vi "GW_Search_id.vi"(8 "error in (no error)":errorcluster, 10 "id":i16, 11 "DBlink":string="Driver={ODBC Driver 17 for SQL Server};Server=localhost\\SQLEXPRESS;Database=ZDX201;UID=labview;PWD=Dsa@54137926") -> (0 "error out":errorcluster, 1 "[glue_data_id]":string, 2 "找到":bool, 3 "取得ID":i16)   [LabVIEW 2019]
uses:
  <vilib>/addons/database/Connection.llb/DB Tools Open Connec (String).vi
  <vilib>/addons/database/Connection.llb/Conn Execute.vi
  <vilib>/addons/database/Recordset.llb/Rec Fetch Recordset Data (R).vi
  <vilib>/addons/database/Recordset.llb/Rec Destroy - Connection.vi
  <vilib>/addons/database/_DB Variant To Data/Database Variant To Data.xnode
  <vilib>/addons/database/NI_Database_API.lvlib
panel:
  out "size(s)":i32
  out "查詢結果":string="SELECT \n      [glue_data_id]\n  FROM [ZDX201].[dbo].[glue_workspace]\n where  [glue_data_id] is not null  and  [id]=0"
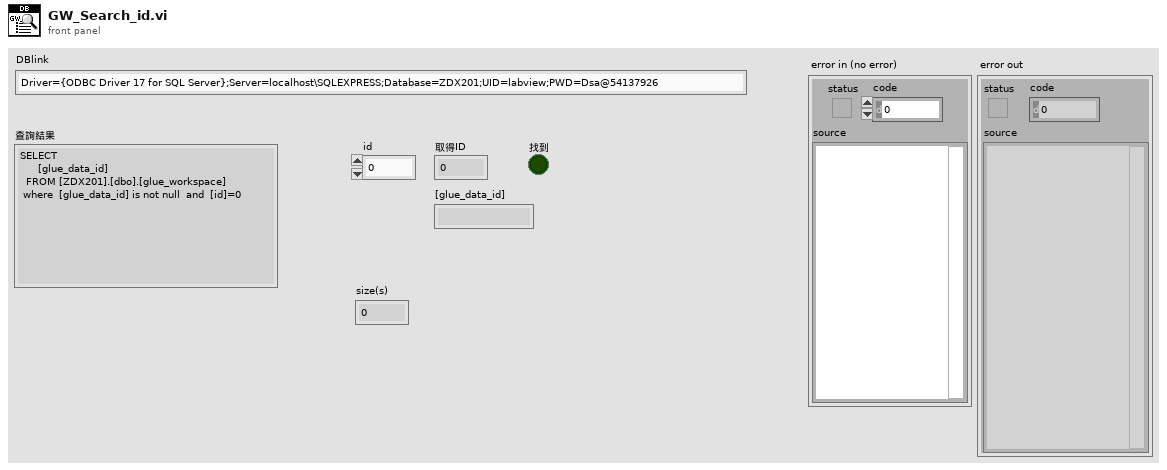
[diagram p1: front panel]
types:
  T1 = typedef "NI_Database_API.lvlib/Conn ObjectReference.ctl" = refnum<k1>
  T2 = typedef "NI_Database_API.lvlib/Rec ObjectReference.ctl" = refnum<k1>
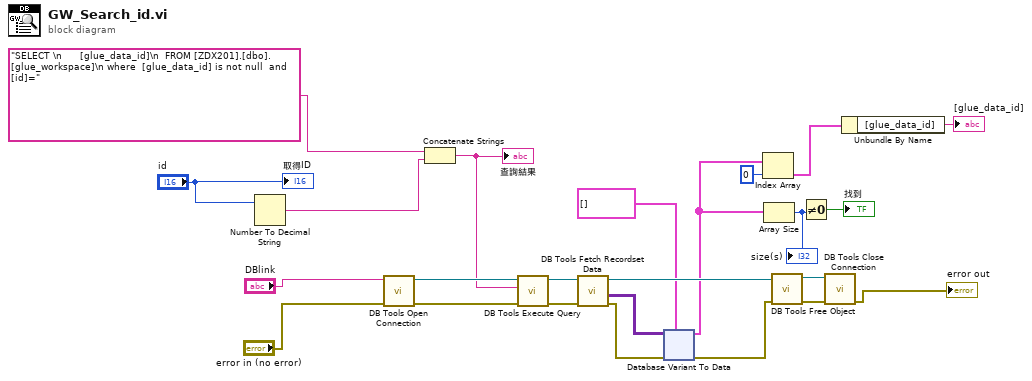
[diagram p0: block diagram]
diagram:
  n1 = Number To Decimal String(number="id") -> (decimal integer string=w8:string)  [unwired: 1 in]
  n2 = call-poly <vilib>:"DB Tools Open Connection.vi"("error in (no error)"="error in (no error)", "connection information"="DBlink") -> ("error out"=w24:errorcluster, "connection reference"=w23:T1)  [unwired: 6 in]
  n3 = Concatenate Strings("SELECT \n      [glue_data_id]\n  FROM [ZDX201].[dbo].[glue_workspace]\n where  [glue_data_id] is not null  and  [id]=", w8) -> (w7:string)
  "查詢結果" <- w7
  n4 = call-poly <vilib>:"DB Tools Execute Query.vi"("error in (no error)"=w24, "SQL query"=w7, "connection reference"=w23) -> ("error out"=w21:errorcluster, "recordset reference"=w22:T2)  [unwired: 5 in]
  n5 = call-poly <vilib>:"DB Tools Fetch Recordset Data.vi"("error in (no error)"=w21, "recordset reference"=w22) -> ("error out"=w16:errorcluster, "recordset data"=w15:variant[][], "recordset reference out"=w17:T2)  [unwired: 3 in]
  n6 = xnode "Database Variant To Data"("database variant"=w15, "error in (no error)"=w16, "type"=cluster{"[glue_data_id]":string}[] [] ("Workplace: assemble")) -> ("data"=w4:cluster{"[glue_data_id]":string}[], "error out"=w18:errorcluster)
  n7 = Index Array(array=w4, index=0) -> (element=w2:cluster{"[glue_data_id]":string})
  n8 = Array Size(array=w4) -> (size(s)=w6:i32)
  "size(s)" <- w6
  n9 = call-poly <vilib>:"DB Tools Free Object.vi"("error in (no error)"=w18, "recordset reference"=w17) -> ("error out"=w19:errorcluster, "connection reference"=w20:T1)  [unwired: 8 in]
  n10 = Not Equal To 0?(x=w6) -> (x != 0?=→"找到":bool)
  n11 = call <vilib>:"DB Tools Close Connection.vi"("error in (no error)"=w19, "connection reference"=w20) -> ("error out"=→"error out":errorcluster)  [unwired: 5 in]
  n12 = Unbundle By Name(w2) -> ("[glue_data_id]"=→"[glue_data_id]":string)
  "取得ID" <- "id"
